vi "FPDAQtoDAQstrings.vi"(1 "front panel":T1 {"AI Configuration"."AI.Coupling" items=["AC"=10045, "DC"=10050, "GND"=10066]; "Channels: AO"."AO f (Hz)" min=0.001 max=10000.0; "Channels: AO"."AO DC (V)" format="%.3p"; "Channels: AO"."AO Amp (V)" format="%.3p"; "Channels: Lockin"."REF phi (°)" format="%#_3g"}) -> (0 "front panel (DAQmx strings)":T22 {"AI Configuration"."AI.Coupling" items=["AC"=10045, "DC"=10050, "GND"=10066]; "Channels: AO"."AO f (Hz)" min=0.001 max=10000.0; "Channels: AO"."AO DC (V)" format="%.3p"; "Channels: AO"."AO Amp (V)" format="%.3p"; "Channels: Lockin"."REF phi (°)" format="%#_3g"})   [LabVIEW 2016, in "LockinDAQ.lvclass"]
uses:
  LockinDAQ.lvclass
  Typedefs/446xAO-enum.ctl
  Typedefs/AI.coupling-enum.ctl
  Typedefs/446xAI-enum.ctl
  Typedefs/AO-cluster.ctl
  Typedefs/AO_Amp-array.ctl
  Typedefs/AO_DC-array.ctl
  Typedefs/AO_f-array.ctl
  Typedefs/AO_phi-array.ctl
  Typedefs/Function-array.ctl
  Typedefs/Function-enum.ctl
  Typedefs/REF-cluster.ctl
  Typedefs/REF_f-array.ctl
  Typedefs/REF_phi-array.ctl
  Typedefs/DAQType-enum.ctl
  Typedefs/AmplifierType-enum.ctl
  Typedefs/Front Panel Cluster.ctl
  Typedefs/AO.config(UI)-array.ctl
  Typedefs/AO.config(UI)-cluster.ctl
  Typedefs/AI.config(UI)-array.ctl
  Typedefs/AI.config(UI)-cluster.ctl
  Typedefs/Cal Info - Cluster.ctl
panel:
  # "1"
  # "2"
  # "3"
  # "4"
  # "5"
  # "6"
  # "7"
  # "8"
  # "1"
  # "2"
  # "3"
  # "4"
  # "5"
  # "6"
  # "7"
  # "8"
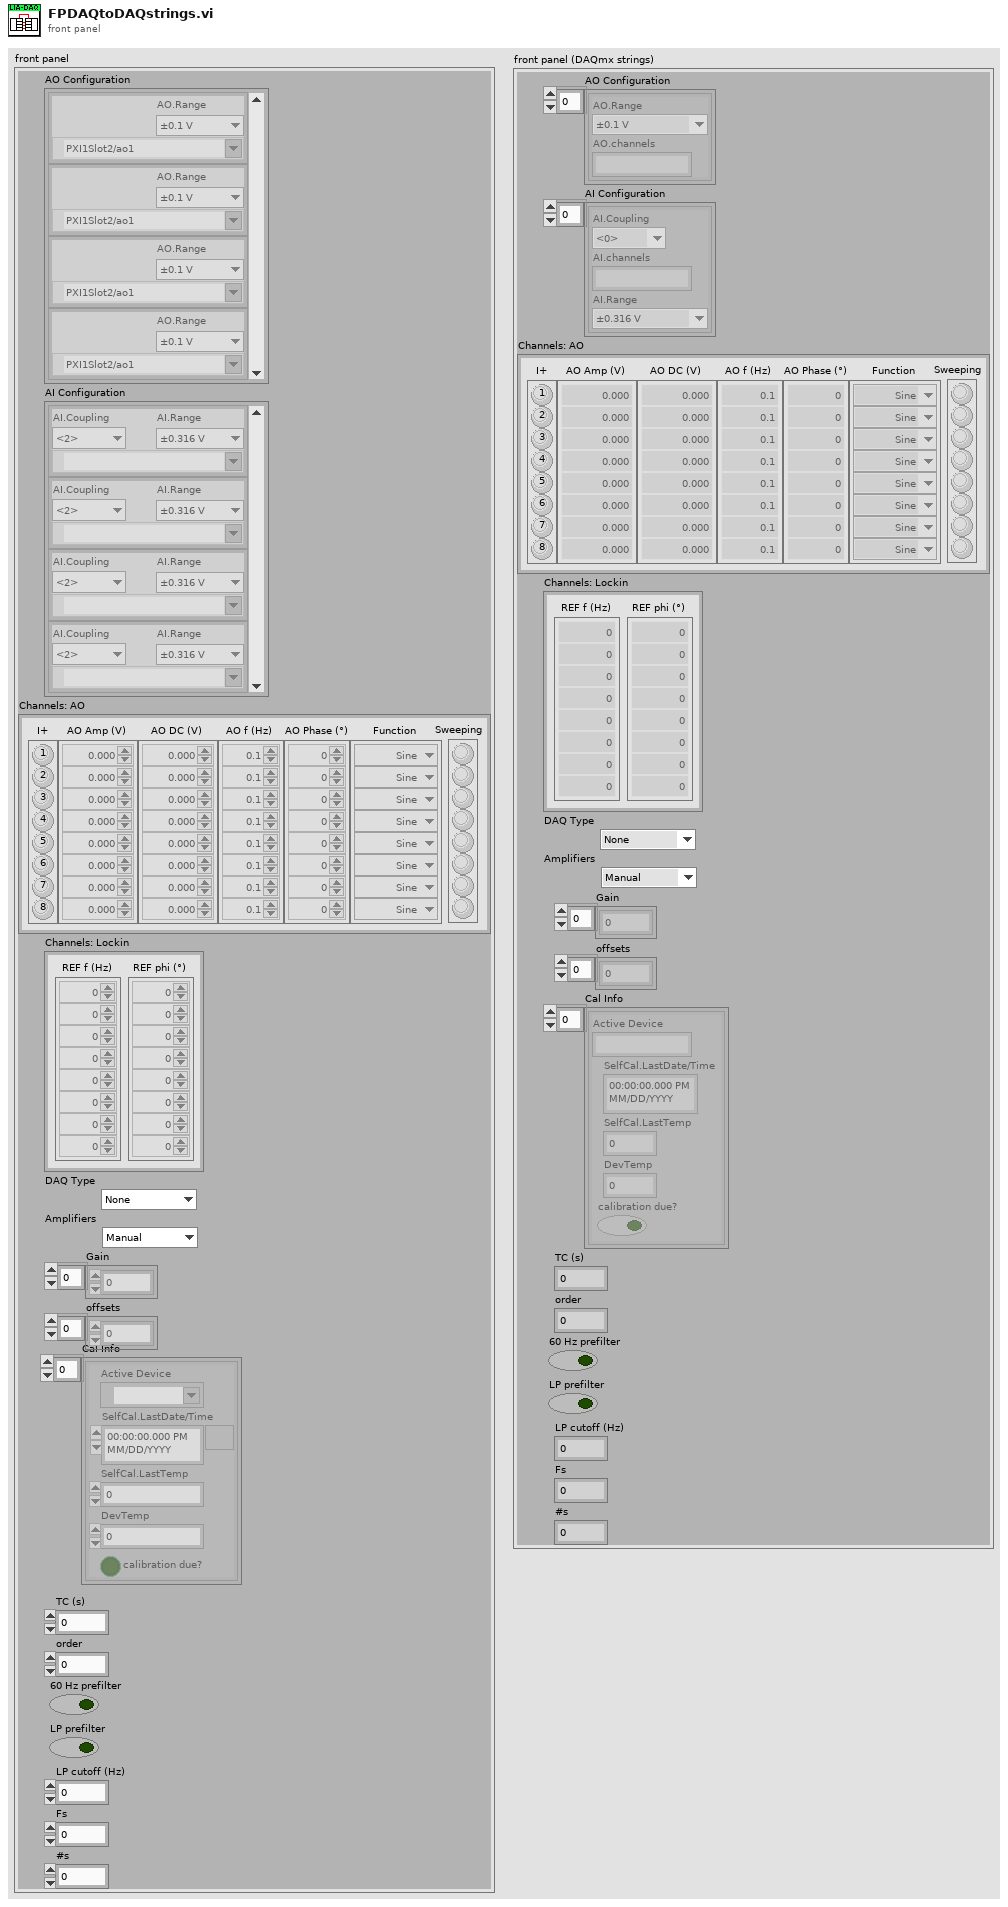
[diagram p1: front panel]
types:
  T1 = typedef "LockinDAQ.lvclass/Front Panel Cluster.ctl" = cluster{"AO Configuration":T2, "AI Configuration":T5, "Channels: AO":T9, "Channels: Lockin":T16, "DAQ Type":T19, "Amplifiers":T20, "Gain":dbl[], "offsets":dbl[], "Cal Info":T21[], "TC (s)":dbl, "order":i32, "60 Hz prefilter":bool, "LP prefilter":bool, "LP cutoff (Hz)":dbl, "Fs":i32, "#s":i32}
  T2 = typedef "LockinDAQ.lvclass/AO.config(UI)-array.ctl" = T3[]
  T3 = typedef "LockinDAQ.lvclass/AO.config(UI)-cluster.ctl" = cluster{"AO.Range":T4, "AO.channels":tag}
  T4 = typedef "LockinDAQ.lvclass/446xAO-enum.ctl" = enum16{"±0.1 V", "±1.0 V", "±10.0 V"}
  T5 = typedef "LockinDAQ.lvclass/AI.config(UI)-array.ctl" = T6[]
  T6 = typedef "LockinDAQ.lvclass/AI.config(UI)-cluster.ctl" = cluster{"AI.Coupling":T7, "AI.channels":tag, "AI.Range":T8}
  T7 = typedef "LockinDAQ.lvclass/AI.coupling-enum.ctl" = u16
  T8 = typedef "LockinDAQ.lvclass/446xAI-enum.ctl" = enum16{"±0.316 V", "±1.00 V", "±3.16 V", "±10.0 V", "±31.6 V", "±42.4 V"}
  T9 = typedef "LockinDAQ.lvclass/AO-cluster.ctl" = cluster{"AO Amp (V)":T10, "AO DC (V)":T11, "AO f (Hz)":T12, "AO Phase (°)":T13, "Function":T14, "I+":bool[], "Sweeping":bool[]}
  T10 = typedef "LockinDAQ.lvclass/AO_Amp-array.ctl" = dbl[]
  T11 = typedef "LockinDAQ.lvclass/AO_DC-array.ctl" = dbl[]
  T12 = typedef "LockinDAQ.lvclass/AO_f-array.ctl" = dbl[]
  T13 = typedef "LockinDAQ.lvclass/AO_phi-array.ctl" = dbl[]
  T14 = typedef "LockinDAQ.lvclass/Function-array.ctl" = T15[]
  T15 = typedef "LockinDAQ.lvclass/Function-enum.ctl" = enum16{"Sine", "Triangle", "Square", "Sawtooth"}
  T16 = typedef "LockinDAQ.lvclass/REF-cluster.ctl" = cluster{"REF f (Hz)":T17, "REF phi (°)":T18}
  T17 = typedef "LockinDAQ.lvclass/REF_f-array.ctl" = dbl[]
  T18 = typedef "LockinDAQ.lvclass/REF_phi-array.ctl" = dbl[]
  T19 = typedef "LockinDAQ.lvclass/DAQType-enum.ctl" = enum16{"None", "USB 4431", "PXI 446x"}
  T20 = typedef "LockinDAQ.lvclass/AmplifierType-enum.ctl" = enum16{"Manual", "Krohn Hite", "Femto"}
  T21 = typedef "LockinDAQ.lvclass/Cal Info - Cluster.ctl" = cluster{"Active Device":tag, "SelfCal.LastDate/Time":timestamp, "SelfCal.LastTemp":dbl, "DevTemp":dbl, "calibration due?":bool}
  T22 = cluster{"AO Configuration":cluster{"AO.Range":T4, "AO.channels":string}[], "AI Configuration":cluster{"AI.Coupling":T7, "AI.channels":string, "AI.Range":T8}[], "Channels: AO":T9, "Channels: Lockin":T16, "DAQ Type":T19, "Amplifiers":T20, "Gain":dbl[], "offsets":dbl[], "Cal Info":cluster{"Active Device":string, "SelfCal.LastDate/Time":timestamp, "SelfCal.LastTemp":dbl, "DevTemp":dbl, "calibration due?":bool}[], "TC (s)":dbl, "order":i32, "60 Hz prefilter":bool, "LP prefilter":bool, "LP cutoff (Hz)":dbl, "Fs":i32, "#s":i32}
  T23 = cluster{"AI.Coupling":T7, "AI.channels":string, "AI.Range":T8}
  T24 = cluster{"Active Device":string, "SelfCal.LastDate/Time":timestamp, "SelfCal.LastTemp":dbl, "DevTemp":dbl, "calibration due?":bool}
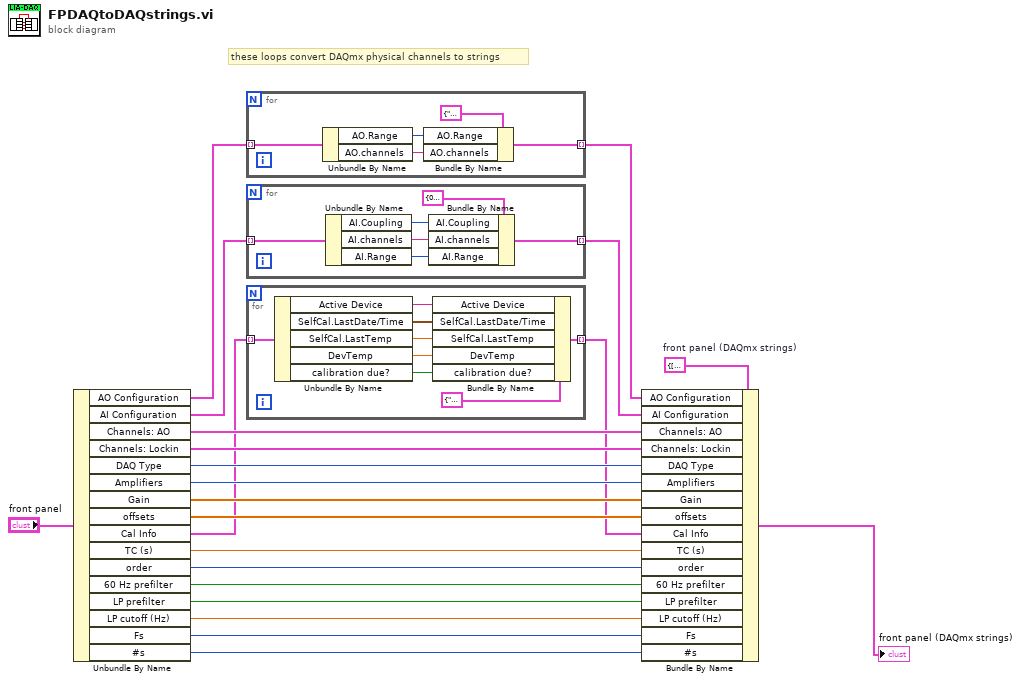
[diagram p0: block diagram]
diagram:
  w22 = T22 {"AO Configuration"=[], "AI Configuration"=[], "Channels: AO"={"AO Amp (V)"=[], "AO DC (V)"=[], "AO f (Hz)"=[], "AO Phase (°)"=[], "Function"=[], "I+"=[], "Sweeping"=[]}, "Channels: Lockin"={"REF f (Hz)"=[], "REF phi (°)"=[]}, "DAQ Type"=enum."None", "Amplifiers"=enum."Manual", "Gain"=[], "offsets"=[], "Cal Info"=[], "TC (s)"=0.0, "order"=0, "60 Hz prefilter"=FALSE, "LP prefilter"=FALSE, "LP cutoff (Hz)"=0.0, "Fs"=0, "#s"=0}  # front panel (DAQmx strings)
  # "these loops convert DAQmx physical channels to strings"
  n1 = Unbundle By Name("front panel") -> ("AO Configuration"=w20:T2, "AI Configuration"=w19:T5, "Channels: AO"=w18:T9, "Channels: Lockin"=w17:T16, "DAQ Type"=w16:T19, "Amplifiers"=w15:T20, "Gain"=w14:dbl[], "offsets"=w13:dbl[], "Cal Info"=w12:T21[], "TC (s)"=w11:dbl, "order"=w10:i32, "60 Hz prefilter"=w9:bool, "LP prefilter"=w8:bool, "LP cutoff (Hz)"=w7:dbl, "Fs"=w6:i32, "#s"=w5:i32)
  n2 = for {
    tunnel: w20 -> [w27] mode=indexing
    tunnel: [w25] -> w2 mode=indexing
    n3 = Unbundle By Name(w27) -> ("AO.Range"=w26:T4, "AO.channels"=w23:tag)
    n4 = Bundle By Name(cluster=cluster{"AO.Range":T4, "AO.channels":string} {"AO.Range"=enum."±0.1 V", "AO.channels"=""}, "AO.Range"=w26, "AO.channels"=w23) -> (w25:cluster{"AO.Range":T4, "AO.channels":string})
  }
  n5 = for {
    tunnel: w19 -> [w33] mode=indexing
    tunnel: [w32] -> w3 mode=indexing
    n6 = Unbundle By Name(w33) -> ("AI.Coupling"=w28:T7, "AI.channels"=w29:tag, "AI.Range"=w30:T8)
    n7 = Bundle By Name(cluster=T23 {"AI.Coupling"=0, "AI.channels"="", "AI.Range"=enum."±0.316 V"}, "AI.Coupling"=w28, "AI.channels"=w29, "AI.Range"=w30) -> (w32:T23)
  }
  n8 = for {
    tunnel: w12 -> [w40] mode=indexing
    tunnel: [w41] -> w4 mode=indexing
    n9 = Unbundle By Name(w40) -> ("Active Device"=w34:tag, "SelfCal.LastDate/Time"=w35:timestamp, "SelfCal.LastTemp"=w36:dbl, "DevTemp"=w37:dbl, "calibration due?"=w38:bool)
    n10 = Bundle By Name(cluster=T24 {"Active Device"="", "SelfCal.LastDate/Time"=timestamp(0 s since 1904-01-01), "SelfCal.LastTemp"=0.0, "DevTemp"=0.0, "calibration due?"=FALSE}, "Active Device"=w34, "SelfCal.LastDate/Time"=w35, "SelfCal.LastTemp"=w36, "DevTemp"=w37, "calibration due?"=w38) -> (w41:T24)
  }
  n11 = Bundle By Name(cluster=w22, "AO Configuration"=w2, "AI Configuration"=w3, "Channels: AO"=w18, "Channels: Lockin"=w17, "DAQ Type"=w16, "Amplifiers"=w15, "Gain"=w14, "offsets"=w13, "Cal Info"=w4, "TC (s)"=w11, "order"=w10, "60 Hz prefilter"=w9, "LP prefilter"=w8, "LP cutoff (Hz)"=w7, "Fs"=w6, "#s"=w5) -> (→"front panel (DAQmx strings)":T22)
